vi "QueueSave.vi"(4 "error in (no error)":errorcluster, 5 "Write To Spreadsheet":bool, 6 "Data In":dbl[](array[numeric]), 7 "Save Data?":bool) -> (0 "error out":errorcluster, 2 "Total Saved Time (s)":dbl, 3 "Segments Saved":u32)   [LabVIEW 2023]
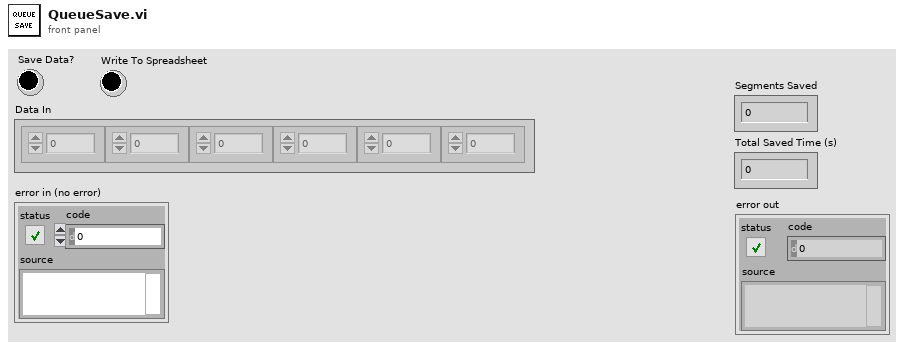
[diagram p1: front panel]
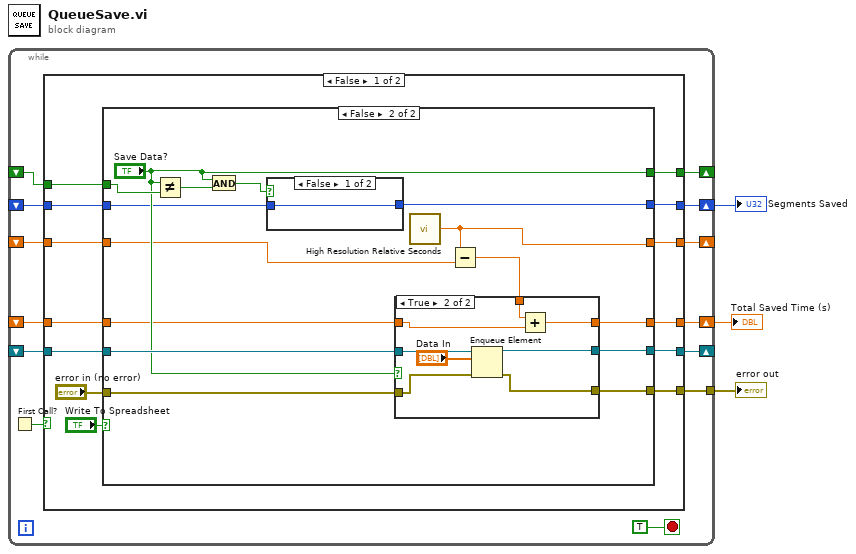
[diagram p0: block diagram]
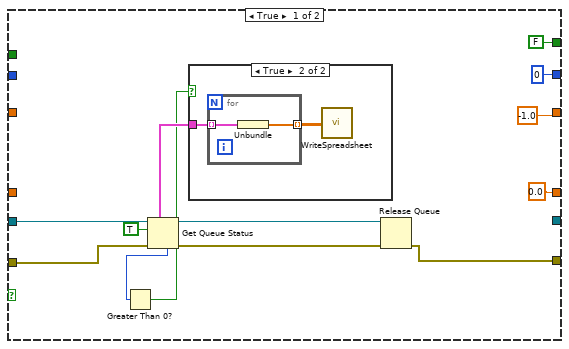
[diagram p2: hidden frame]
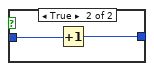
[diagram p4: hidden frame]
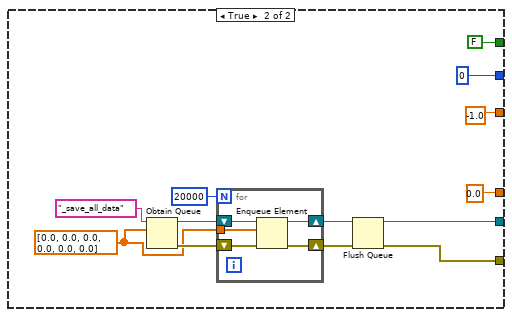
[diagram p6: hidden frame]
diagram:
  n1 = while {
    shift-right: [w14] -> _
    shift-left: _ -> [w13]
    tunnel: [w12] -> w3
    shift-right: [w11] -> _
    shift-left: _ -> [w8]
    shift-right: [w10] -> w2
    shift-left: _ -> [w7]
    shift-right: [w9] -> w1
    shift-left: _ -> [w6]
    shift-right: [w5] -> _
    shift-left: _ -> [w4]
    stop <- TRUE stop-if-true
    n2 = First Call?() -> (First Call?: T/F=w15:bool)
    n3 = case shown="False" w15 {
      tunnel: [w28 w81] -> w14
      tunnel: w13 -> [w29 _]
      tunnel: [w27 w80] -> w12
      tunnel: [w21 FALSE] -> w11
      tunnel: [w20 u32 0 ("Segments Saved")] -> w10
      tunnel: [w18 0.0 ("Segments Saved")] -> w9
      tunnel: w8 -> [w24 _]
      tunnel: w7 -> [w23 _]
      tunnel: w6 -> [w22 _]
      tunnel: [w17 -1.0 ("Segments Saved")] -> w5
      tunnel: w4 -> [w19 _]
      frame False {
        n4 = case shown="False" "Write To Spreadsheet" {
          tunnel: w29 -> [w42 w61]
          tunnel: [_ w60] -> w28
          tunnel: [w38 w59] -> w27
          tunnel: "error in (no error)" -> [w37 w58]
          tunnel: w24 -> [_ w57]
          tunnel: w23 -> [_ w53]
          tunnel: w22 -> [_ w51]
          tunnel: [FALSE ("Save Data?") "Save Data?"] -> w21
          tunnel: [u32 0 ("Segments Saved") w52] -> w20
          tunnel: w19 -> [_ w48]
          tunnel: [0.0 ("Segments Saved") w50] -> w18
          tunnel: [-1.0 ("Segments Saved") w47] -> w17
          frame True {
            n5 = Get Queue Status(queue=w42, return elements? (F)=TRUE, error in (no error)=w37) -> (queue out=w41:refnum<queue>, error out=w39:errorcluster, # elements in queue=w35:i32, elements=w36:cluster{dbl[]}[])  [unwired: 4 out]
            n6 = Greater Than 0?(x=w35) -> (x > 0?=w34:bool)
            n7 = case shown="True" w34 {
              tunnel: w36 -> [_ w44]
              frame False {
              }
              frame True {
                n8 = for {
                  tunnel: w44 -> [w46] mode=indexing
                  tunnel: [w45] -> w43 mode=indexing
                  n9 = Unbundle(w46) -> (w45:dbl[])
                }
                n10 = call "WriteSpreadsheet.vi"("2-d array of\nnumbers"=w43) -> ()
              }
            }
            n11 = Release Queue(queue=w41, error in (no error)=w39) -> (error out=w38:errorcluster)  [unwired: 1 in, 2 out]
          }
          frame False {
            n12 = Not Equal?(x="Save Data?", y=w57) -> (x != y?=w56:bool)
            n13 = And(x="Save Data?", y=w56) -> (x .and. y?=w54:bool)
            n14 = case shown="False" w54 {
              tunnel: w53 -> [w62 w64]
              tunnel: [w62 w63] -> w52
              frame False {
              }
              frame True {
                n15 = Increment(x=w64) -> (x+1=w63:u32)
              }
            }
            n16 = call <vilib>:"High Resolution Relative Seconds.vi"() -> ("relative seconds"=w47:dbl)
            n17 = Subtract(x=w47, y=w48) -> (x-y=w49:dbl)
            n18 = case shown="True" "Save Data?" {
              tunnel: w61 -> [w67 w75]
              tunnel: [w67 w74] -> w60
              tunnel: [w66 w72] -> w59
              tunnel: w58 -> [w66 w71]
              tunnel: w51 -> [w65 w69]
              tunnel: [w65 w70] -> w50
              tunnel: w49 -> [_ w68]
              frame False {
              }
              frame True {
                n19 = Enqueue Element(queue=w75, element="Data In", error in (no error)=w71) -> (queue out=w74:refnum<queue>, error out=w72:errorcluster)  [unwired: 1 in, 1 out]
                n20 = Add(x=w68, y=w69) -> (x+y=w70:dbl)
              }
            }
          }
        }
      }
      frame True {
        w83 = dbl[] [0.0, 0.0, 0.0, 0.0, 0.0, 0.0]
        n21 = Obtain Queue(name (unnamed)="_save_all_data", element data type=w83) -> (queue out=w88:refnum<queue>, error out=w87:errorcluster)  [unwired: 3 in, 1 out]
        n22 = for {
          N: 20000 -> [_]
          tunnel: w83 -> [w92]
          shift-right: [w89] -> w85
          shift-left: w88 -> [w93]
          shift-right: [w90] -> w86
          shift-left: w87 -> [w91]
          n23 = Enqueue Element(queue=w93, element=w92, error in (no error)=w91) -> (queue out=w89:refnum<queue>, error out=w90:errorcluster)  [unwired: 1 in, 1 out]
        }
        n24 = Flush Queue(queue=w85, error in (no error)=w86) -> (queue out=w81:refnum<queue>, error out=w80:errorcluster)  [unwired: 1 out]
      }
    }
  }
  "error out" <- w3
  "Segments Saved" <- w2
  "Total Saved Time (s)" <- w1
